vi "CloseLib.vi"(0 "error in (no error)":errorcluster) -> (1 "GX_STATUS":i32, 2 "error out":errorcluster)   [LabVIEW 2016, in "GxLVLib.lvlib"]
uses:
  GxLVLib.lvlib
  GxIAPI.dll
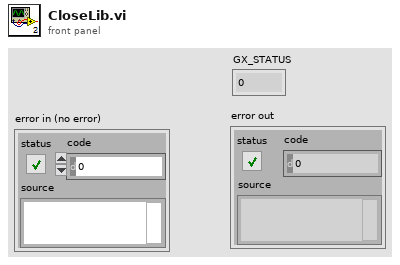
[diagram p1: front panel]
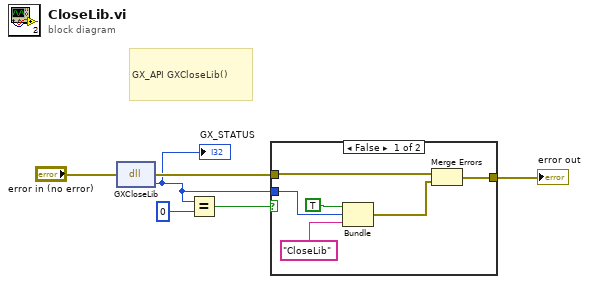
[diagram p0: block diagram]
diagram:
  # "GX_API GXCloseLib()"
  n1 = dll-call lib="GxIAPI.dll" fn="GXCloseLib"(error in="error in (no error)") -> (error out=w4:errorcluster, "GX_STATUS"=w1:i32)  [unwired: 2 in, 1 out]
  "GX_STATUS" <- w1
  n2 = Equal?(x=w1, y=0) -> (x = y?=w2:bool)
  n3 = case shown="False" w2 {
    tunnel: w4 -> [w12 w13]
    tunnel: [w11 w13] -> w5
    tunnel: w1 -> [w9 _]
    frame False {
      n4 = Bundle(TRUE, "GX_STATUS"=w9, "CloseLib") -> (w10:cluster{bool, "GX_STATUS":i32, string})  [unwired: 1 in]
      n5 = Merge Errors(w12, w10) -> (w11:errorcluster)
    }
    frame True {
    }
  }
  "error out" <- w5
